vi "dscCancelOp.vi"(8 "error in":errorcluster, 11 "board":i16) -> (0 "error out":errorcluster, 3 "boardOut":i16)   [LabVIEW 2011, in "Diamond Universal Driver.lvlib"]
doc: "Terminate all currently running interrupt operations on the board. If there is no currently running interrupt operation then the function will return the error DE_NONE_IN_PROGRESS."
uses:
  Diamond Universal Driver.lvlib
  Controls/error codes.ctl
  Instruments/WL OPC/Support/dlls/dscud.dll
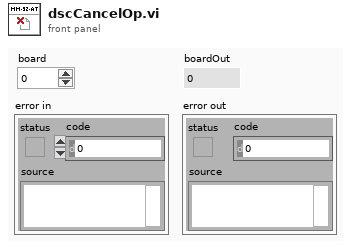
[diagram p1: front panel]
types:
  T1 = typedef "Diamond Universal Driver.lvlib/error codes.ctl" = enum8{"DE_NONE", "DE_HW_FAILURE", "DE_SW_FAILURE", "DE_HW_NOT_SUPPORTED", "DE_SW_NOT_SUPPORTED", "DE_INVALID_PARM", "DE_ALTERNATE_IN_PROGRESS", "DE_NONE_IN_PROGRESS", "DE_BUFFER_ROLLOVER", "DE_INVALID_ERROR_CODE", "DE_ALREADY_PAUSED", "DE_OVERFLOW", "DE_INVALID_FUNC", "DE_DSCUDH_INVALID", "DE_INVALID_BOARD", "DE_BOARD_LIMIT_REACHED", "DE_BOARD_BUSY", "DE_INVALID_WINDRVR_HANDLE", "DE_INVALID_WINDRVR_VERSION", "DE_BAD_WINDRVR_BOARD_INIT", "DE_OPERATION_TIMED_OUT", "DE_INVALID_WINDRVR_KP", "DE_THREAD_FAILURE"}
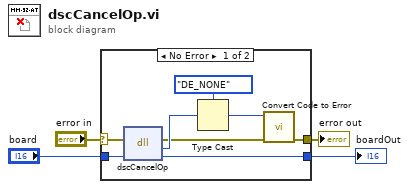
[diagram p0: block diagram]
diagram:
  n1 = case shown="No Error" "error in" {
    selector: "error in" -> [w11 w14]
    tunnel: "board" -> [w12 w13]
    tunnel: [w9 w13] -> w2
    tunnel: [w5 w14] -> w1
    frame No Error {
      n2 = dll-call lib="C:/Users/mrichardson/Documents/Web Based Version Control SW/Instruments/WL OPC/Support/dlls/dscud.dll" fn="dscCancelOp"(error in=w11, "board"=w12) -> (error out=w6:errorcluster, "error"=w10:u8, "board"=w9:i16)  [unwired: 2 in, 1 out]
      n3 = Type Cast(type=error_codes."DE_NONE" ("error codes"), x=w10) -> (*(type *) &x=w8:T1)
      n4 = call "Convert Code to Error.vi"("error in"=w6, "error codes"=w8) -> ("error out"=w5:errorcluster)  [unwired: 9 in]
    }
    frame Error {
    }
  }
  "error out" <- w1
  "boardOut" <- w2
